vi "Update Mecanum Wheel FP Values.vi"(4 "angle mode":T1=1 items=["Degrees", "Radians"], 8 "error in (no error)":errorcluster, 10 "fp refs":T2, 11 "wheels in":refnum<class "NI_Robotics_Wheel.lvclass">[](array[class])) -> (0 "error out":errorcluster, 2 "dup fp refs":T2, 3 "wheels out":refnum<class "NI_Robotics_Wheel.lvclass">[](array[class]))   [LabVIEW 2017, in "NI_Robotics_Configure Steering Frame.lvlib" / "User Defined Frame Subpanel.lvlib"]
uses:
  <vilib>/robotics/Dialog/Configure Steering Frame/User Defined Frame Subpanel/User Defined Frame Subpanel.lvlib
  <vilib>/robotics/Dialog/Configure Steering Frame/User Defined Frame Subpanel/FP Refs.ctl
  <vilib>/robotics/Steering/Wheel/NI_Robotics_Wheel.lvclass
  <vilib>/robotics/Dialog/Configure Steering Frame/Angle Mode.ctl
  <vilib>/robotics/Steering/Wheel/Get Mecanum Wheel Information.vi
  <vilib>/robotics/Dialog/Configure Steering Frame/NI_Robotics_Configure Steering Frame.lvlib
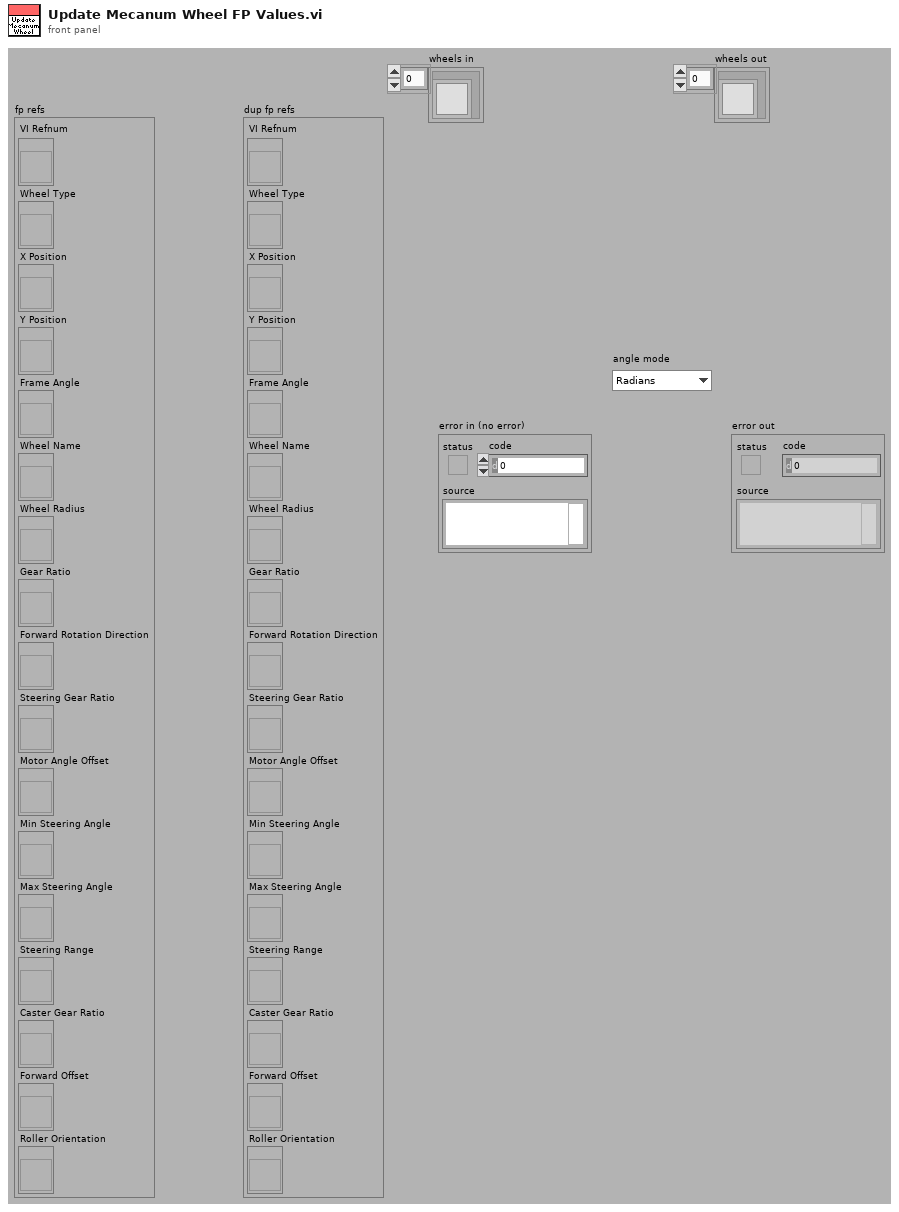
[diagram p1: front panel]
types:
  T1 = typedef "NI_Robotics_Configure Steering Frame.lvlib/Angle Mode.ctl" = u16
  T2 = typedef "NI_Robotics_Configure Steering Frame.lvlib/User Defined Frame Subpanel.lvlib/FP Refs.ctl" = cluster{"VI Refnum":refnum<vi>, "Wheel Type":refnum<vi>, "X Position":refnum<vi>, "Y Position":refnum<vi>, "Frame Angle":refnum<vi>, "Wheel Name":refnum<vi>, "Wheel Radius":refnum<vi>, "Gear Ratio":refnum<vi>, "Forward Rotation Direction":refnum<vi>, "Steering Gear Ratio":refnum<vi>, "Motor Angle Offset":refnum<vi>, "Min Steering Angle":refnum<vi>, "Max Steering Angle":refnum<vi>, "Steering Range":refnum<vi>, "Caster Gear Ratio":refnum<vi>, "Forward Offset":refnum<vi>, "Roller Orientation":refnum<vi>}
  T3 = typedef "NI_Robotics_Mecanum Wheel.lvclass/Roller Orientation.ctl" = u16
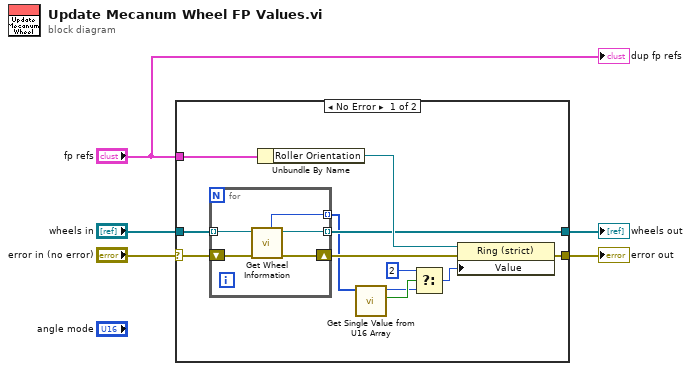
[diagram p0: block diagram]
diagram:
  n1 = case shown="No Error" "error in (no error)" {
    selector: "error in (no error)" -> [w16 w23]
    tunnel: [w11 w23] -> w5
    tunnel: "wheels in" -> [w17 w24]
    tunnel: [w12 w24] -> w2
    tunnel: "fp refs" -> [w15 _]
    frame No Error {
      n2 = for {
        tunnel: w17 -> [w22] mode=indexing
        tunnel: [w19] -> w10 mode=indexing
        tunnel: [w18] -> w12 mode=indexing
        shift-right: [w20] -> w14
        shift-left: w16 -> [w21]
        n3 = call-poly <vilib>:"Get Wheel Information.vi"("error in (no error)"=w21, "wheel in"=w22) -> ("error out"=w20:errorcluster, "wheel out"=w18:refnum<class "NI_Robotics_Wheel.lvclass">, "roller orientation"=w19:T3)  [unwired: 4 in, 3 out]
      }
      n4 = Unbundle By Name(w15) -> ("Roller Orientation"=w13:refnum<vi>)
      n5 = call <vilib>:"Get Single Value from U16 Array.vi"("values"=w10) -> ("multiple values"=w8:bool, "single value"=w7:u16)  [unwired: 9 in]
      n6 = Select(t=u16 2, s=w8, f=w7) -> (s? t:f=w9:u16)
      n7 = property class="Ring (strict)"(reference=w13, error in=w14, "Value"=w9) -> (error out=w11:errorcluster)  [unwired: 1 out]
    }
    frame Error {
    }
  }
  "error out" <- w5
  "wheels out" <- w2
  "dup fp refs" <- "fp refs"
